vi "_wmg_updateItemConValue.vi"(1 "Values":string[](array[string]), 2 "Items":string[](array[string])) -> (0 "Output":string)   [LabVIEW 2011]
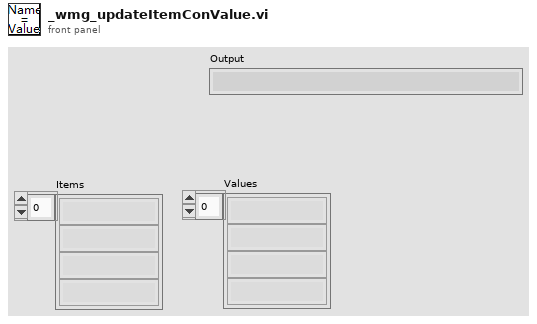
[diagram p1: front panel]
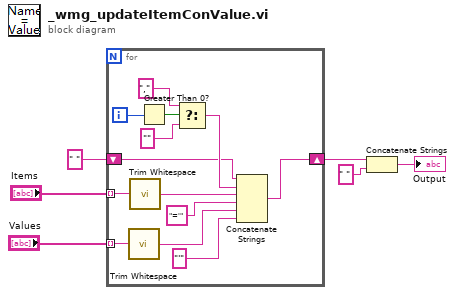
[diagram p0: block diagram]
diagram:
  n1 = for {
    tunnel: "Items" -> [w19] mode=indexing
    tunnel: "Values" -> [w18] mode=indexing
    shift-right: [w7] -> w3
    shift-left: " " -> [w8]
    i -> [w17]
    n2 = call <vilib>:"Trim Whitespace.vi"("string"=w18) -> ("trimmed string"=w11:string)  [unwired: 1 in]
    n3 = call <vilib>:"Trim Whitespace.vi"("string"=w19) -> ("trimmed string"=w13:string)  [unwired: 1 in]
    n4 = Greater Than 0?(x=w17) -> (x > 0?=w16:bool)
    n5 = Select(t=",", s=w16, f="") -> (s? t:f=w9:string)
    n6 = Concatenate Strings(w8, w9, w13, "='", w11, "'") -> (w7:string)
  }
  n7 = Concatenate Strings(w3, " " ("字符串")) -> (→"Output":string)
